vi "x502_err_sub.vi"(1 "Error code":i32, 2 "error in (no error)":errorcluster, 3 "Error descr":string) -> (0 "error out":errorcluster)   [LabVIEW 2018]
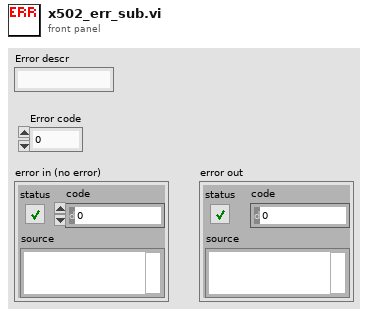
[diagram p1: front panel]
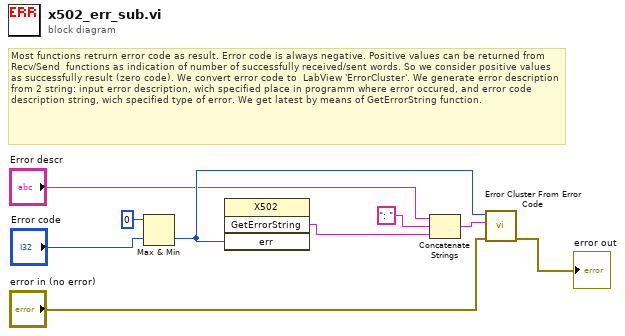
[diagram p0: block diagram]
diagram:
  # "Most functions retrurn error code as result. Error code is always negative. Positive values can be returned from Recv/Send  functions as indication of number of successfully received/sent words. So we consider positive values as successfully result (zero code). We convert error code to  LabView 'ErrorCluster'. We generate error description from 2 string: input error description, wich specified place in programm where error occured, and error code description string, wich specified type of error. We get latest by means of GetErrorString function."
  n1 = Max & Min(x=0, y="Error code") -> (min(x,y)=w7:i32)  [unwired: 1 out]
  n2 = invoke class="X502" method="GetErrorString"("err"=w7) -> ("GetErrorString"=w1:string)  [unwired: 3 in, 3 out]
  n3 = Concatenate Strings("Error descr", ": ", w1) -> (w9:string)
  n4 = call <vilib>:"Error Cluster From Error Code.vi"("error in (no error)"="error in (no error)", "error message (\"\")"=w9, "error code (0)"=w7) -> ("error out"=→"error out":errorcluster)  [unwired: 6 in]
